vi "Board Listing.vi"(8 "error in":errorcluster, 10 "desired port":string) -> (0 "error out":errorcluster, 2 "Array":string[][](array[string]), 3 "Arduino":T1)   [LabVIEW 2022 SP3]
uses:
  ArduinoCtrl.ctl
  9c1b3983-c7ab-5c40-aa67-b4885e2fcccb.vi
  <vilib>/Utility/error.llb/Trim Whitespace One-Sided.vi
  <vilib>/Comparison/Equal/Equal Functor/Equal Functor.lvclass
panel:
  out "standard error":string
  out "Table Control":string[][](table)
  out "String":string
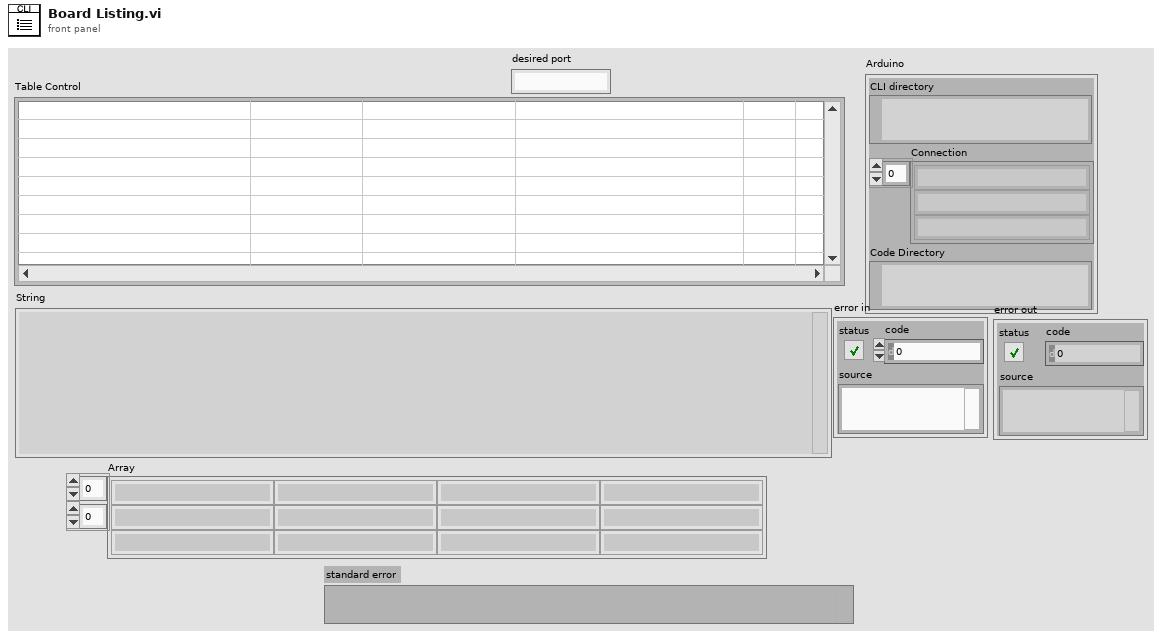
[diagram p1: front panel]
types:
  T1 = typedef "ArduinoCtrl.ctl" = cluster{"CLI directory":path, "Connection":string[], "Code Directory":path}
  T2 = typedef "Preferences.ctl" = cluster{"python":string, "arduino CLI":path, "pythonCodes":cluster{"pythonCode":path, "Color":u32}[], "FontSize":u8, "Text Colors":cluster{"Quote":u32, "function":u32, "Python":u32, "Comment":u32, "Triple Quote":u32, "Text":u32}, "SSH Logins":cluster{"IP Address":string, "Username":string, "password":string}[], "packet size":u8}
  T3 = cluster{"arduino CLI":path, string[], "appended path":path}
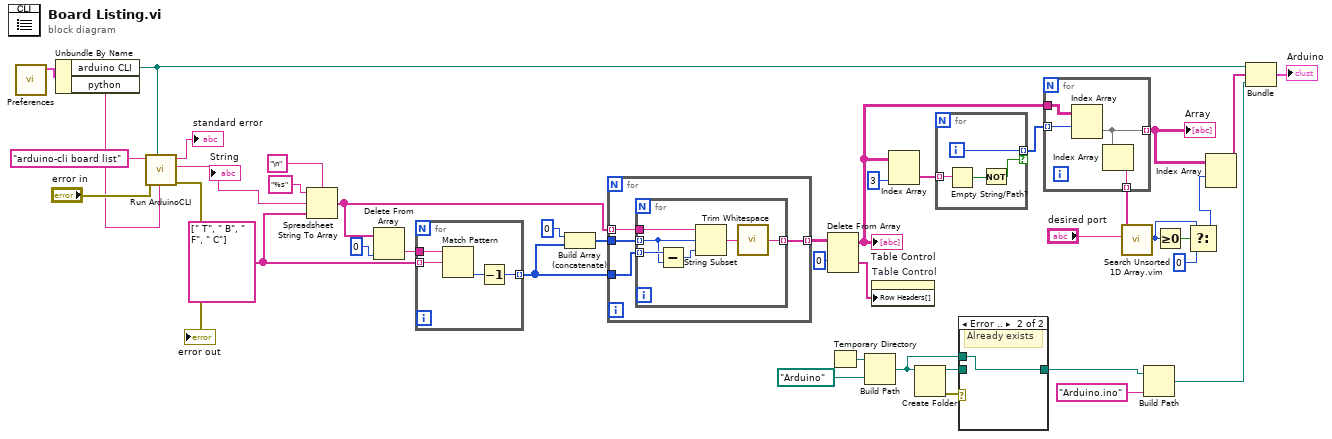
[diagram p0: block diagram]
diagram:
  w37 = string[] [" T", " B", " F", " C"] ("Table Control")
  n1 = call "Preferences.vi"() -> ("Preferences out"=w9:T2)  [unwired: 10 in, 1 out]
  n2 = Unbundle By Name(w9) -> ("arduino CLI"=w8:path, "python"=w2:string)
  n3 = call "Run ArduinoCLI.vi"("Python version"=w2, "working directory"=w8, "error in"="error in", "command line"="arduino-cli board list") -> ("error out"=→"error out":errorcluster, "standard output"=w24:string, "standard error"=→"standard error":string)  [unwired: 5 in]
  "String" <- w24
  n4 = Spreadsheet String To Array(delimiter (Tab)="\n", format string="%s", spreadsheet string=w24, array type (2D Dbl)=w37) -> (array=w32:string[])
  n5 = Delete From Array(array=w32, index=0) -> (deleted portion=w38:string)  [unwired: 1 in, 1 out]
  n6 = for {
    tunnel: w38 -> [w45]
    tunnel: w37 -> [w44] mode=indexing
    tunnel: [w42] -> w35 mode=indexing
    n7 = Match Pattern(string=w45, regular expression=w44) -> (offset past match=w43:i32)  [unwired: 1 in, 3 out]
    n8 = Decrement(x=w43) -> (x-1=w42:i32)
  }
  n9 = Build Array (concatenate)(0, w35) -> (w33:i32[])
  n10 = for {
    tunnel: w32 -> [w49] mode=indexing
    tunnel: w35 -> [w48]
    tunnel: [w47] -> w36 mode=indexing
    tunnel: w33 -> [w46]
    n11 = for {
      tunnel: w49 -> [w55]
      tunnel: w48 -> [w52] mode=indexing
      tunnel: [w50] -> w47 mode=indexing
      tunnel: w46 -> [w51] mode=indexing
      n12 = Subtract(x=w52, y=w51) -> (x-y=w53:i32)
      n13 = String Subset(string=w55, offset (0)=w51, length (rest)=w53) -> (substring=w54:string)
      n14 = call <vilib>:"Trim Whitespace.vi"("string"=w54) -> ("trimmed string"=w50:string)  [unwired: 1 in]
    }
  }
  n15 = Delete From Array(array=w36, index (row)=0) -> (deleted portion=w31:string[], array with subset deleted=w28:string[][])  [unwired: 2 in]
  "Table Control" <- w28
  n16 = Temporary Directory() -> (w7:path)
  n17 = Build Path(base path=w7, name or relative path=path "Arduino") -> (appended path=w1:path)
  n18 = property on="Table Control" class="Tbl (strict)"("Row Headers[]"=w31) -> ()  [unwired: 2 in, 2 out]
  n19 = Index Array(array=w28, index (col)=3 ("disabled index (col)")) -> (element=w29:string[])  [unwired: 1 in]
  n20 = Create Folder(path (use dialog)=w1) -> (created path=w3:path, error out=w5:errorcluster)  [unwired: 2 in, 1 out]
  n21 = for {
    tunnel: w29 -> [w59] mode=indexing
    tunnel: [w58] -> w27 mode=indexing if=w56
    i -> [w58]
    n22 = Empty String/Path?(string/path=w59) -> (empty?=w57:bool)
    n23 = Not(x=w57) -> (.not. x?=w56:bool)
  }
  n24 = case shown="Error .." w5 {
    tunnel: [w60 w61] -> w4
    tunnel: w3 -> [w60 _]
    tunnel: w1 -> [_ w61]
    frame No Error {
    }
    frame Error {
      # "Already exists"
    }
  }
  n25 = for {
    tunnel: w28 -> [w65]
    tunnel: w27 -> [w64] mode=indexing
    tunnel: [w63] -> w22 mode=indexing
    tunnel: [w62] -> w15 mode=indexing
    n26 = Index Array(array=w65, index (row)=w64) -> (element=w63:string[])  [unwired: 1 in]
    n27 = Index Array(array=w63) -> (element=w62:string)  [unwired: 1 in]
  }
  "Array" <- w22
  n28 = call "Search Unsorted 1D Array.vim"("element"="desired port", "unsorted 1D array"=w15) -> ("index of element"=w12:i32)  [unwired: 9 in]
  n29 = Build Path(base path=w4, name or relative path="Arduino.ino") -> (appended path=w18:path)
  n30 = Greater Or Equal To 0?(x=w12) -> (x >= 0?=w13:bool)
  n31 = Select(t=w12, s=w13, f=0) -> (s? t:f=w10:i32)
  n32 = Index Array(array=w22, index (row)=w10) -> (element=w21:string[])  [unwired: 1 in]
  n33 = Bundle("arduino CLI"=w8, w21, "appended path"=w18) -> (→"Arduino":T3)  [unwired: 1 in]
